vi "Recall.vi"(0 "LV MDI in":refnum<class "LV MDI.lvclass">, 5 "XML File Path":path, 7 "Container Refnum":refnum<k24>, 11 "error in (no error)":errorcluster) -> (4 "LV MDI out":refnum<class "LV MDI.lvclass">, 6 "Name[]":string[](array[string]), 15 "error out":errorcluster)   [LabVIEW 2016, in "LV MDI.lvclass"]
uses:
  LV MDI.lvclass
  System.Windows.Forms
  TypeDefs/Data to Save.ctl
  TypeDefs/Set Position.ctl
  example/Example1/Typedef/Environment Selection.ctl
  <vilib>/Utility/xml.llb/Read From XML File(string).vi
  Document/Child Classes/LV Doc/LV Doc.lvclass
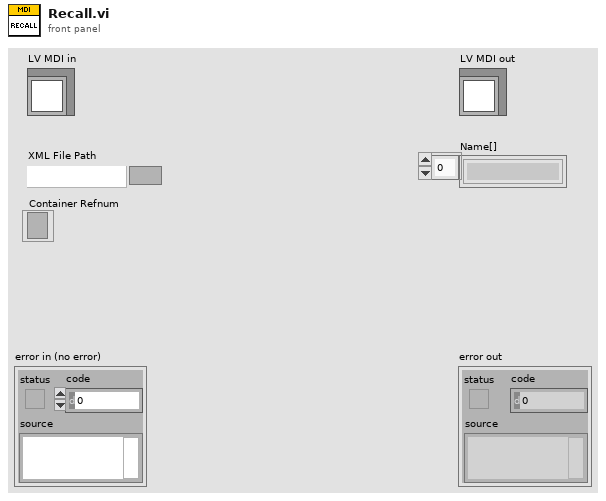
[diagram p1: front panel]
types:
  T1 = typedef "LV MDI.lvclass/Data to Save.ctl" = cluster{"LV MDI out":refnum<class "LV MDI.lvclass">, "Displayed Doc[]":string[], "Position[]":T2[], "Environment Selection":T3}
  T2 = typedef "LV MDI.lvclass/Set Position.ctl" = cluster{"X":i32, "Y":i32, "Width":i32, "Height":i32}
  T3 = typedef "Environment Selection.ctl" = enum16{"RTE", "Dev Environment"}
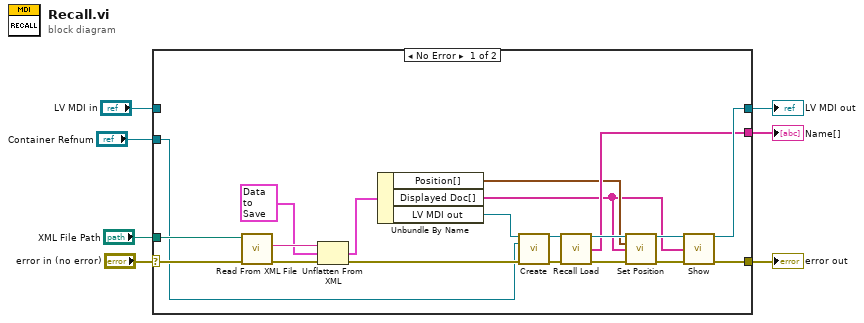
[diagram p0: block diagram]
diagram:
  n1 = case shown="No Error" "error in (no error)" {
    selector: "error in (no error)" -> [w27 w29]
    tunnel: [w14 w29] -> w6
    tunnel: [w11 w28] -> w4
    tunnel: "LV MDI in" -> [_ w28]
    tunnel: "XML File Path" -> [w26 _]
    tunnel: "Container Refnum" -> [w19 _]
    tunnel: [w10 _] -> w1
    frame No Error {
      n2 = call-poly <vilib>:"Read From XML File.vi"("error in (no error)"=w27, "XML File Path"=w26) -> ("error out"=w22:errorcluster, "XML Elements"=w25:string)  [unwired: 7 in, 1 out]
      n3 = Unflatten From XML(xml string=w25, type=T1 {"LV MDI out"=refnum, "Displayed Doc[]"=["Tank.vi Front Panel"], "Position[]"=[{"X"=586, "Y"=186, "Width"=886, "Height"=486}], "Environment Selection"=enum."RTE"} ("Cluster"), error in (no error)=w22) -> (value=w23:T1, error out=w21:errorcluster)
      n4 = Unbundle By Name(w23) -> ("Position[]"=w9:T2[], "Displayed Doc[]"=w8:string[], "LV MDI out"=w20:refnum<class "LV MDI.lvclass">)
      n5 = call "Create.vi"("LV MDI in"=w20, "Panel Reference"=w19, "error in (no error)"=w21) -> ("LV MDI out"=w17:refnum<class "LV MDI.lvclass">, "error out"=w18:errorcluster)  [unwired: 11 in]
      n6 = call "Recall Load.vi"("LV MDI in"=w17, "error in (no error)"=w18) -> ("LV MDI out"=w12:refnum<class "LV MDI.lvclass">, "Name[]"=w10:string[], "error out"=w16:errorcluster)  [unwired: 11 in]
      n7 = call "Set Position.vi"("LV MDI.lvclass"=w12, "Position[]"=w9, "Doc Name[]"=w8, "error in (no error)"=w16) -> ("LV MDI.lvclass"=w13:refnum<class "LV MDI.lvclass">, "error out"=w15:errorcluster)  [unwired: 10 in]
      n8 = call "Show.vi"("LV MDI in"=w13, "Doc Name[]"=w8, "error in (no error)"=w15) -> ("LV MDI out"=w11:refnum<class "LV MDI.lvclass">, "error out"=w14:errorcluster)  [unwired: 11 in]
    }
    frame Error {
    }
  }
  "error out" <- w6
  "LV MDI out" <- w4
  "Name[]" <- w1
